vi "valueToString.vi"(1 "variant":variant) -> (0 "String":string)   [LabVIEW 2015]
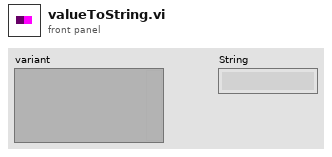
[diagram p1: front panel]
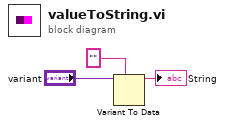
[diagram p0: block diagram]
diagram:
  n1 = Variant To Data(type="", Variant="variant") -> (data=→"String":string)  [unwired: 1 in, 1 out]
